vi "sub_updatepos_fgv.vi"(7 "cmd":enum16{"left", "right", "ini", "read", "write"}(ring), 8 "error in":errorcluster, 10 "pos":dbl(slide) scale=-1.0..1.0, 11 "Target":T1={"Position"=0.0, "Invert"=TRUE} {"Position" min=-0.5 max=0.5 step=0.1 format="%.2g"}) -> (0 "error out":errorcluster, 3 "Target_out":T1={"Position"=0.5, "Invert"=FALSE} {"Position" min=-0.5 max=0.5 step=0.1 format="%.2g"})   [LabVIEW 2018]
uses:
  Model/Target.ctl
  Global_val.vi
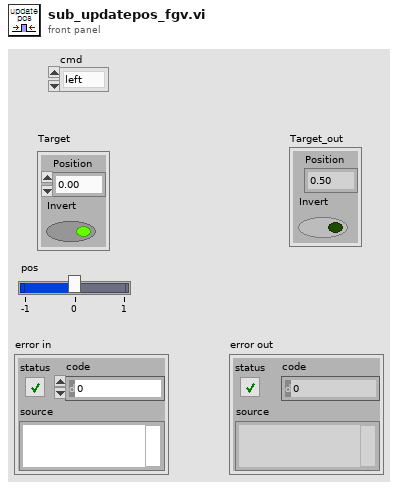
[diagram p1: front panel]
types:
  T1 = typedef "Target.ctl" = cluster{"Position":dbl, "Invert":bool}
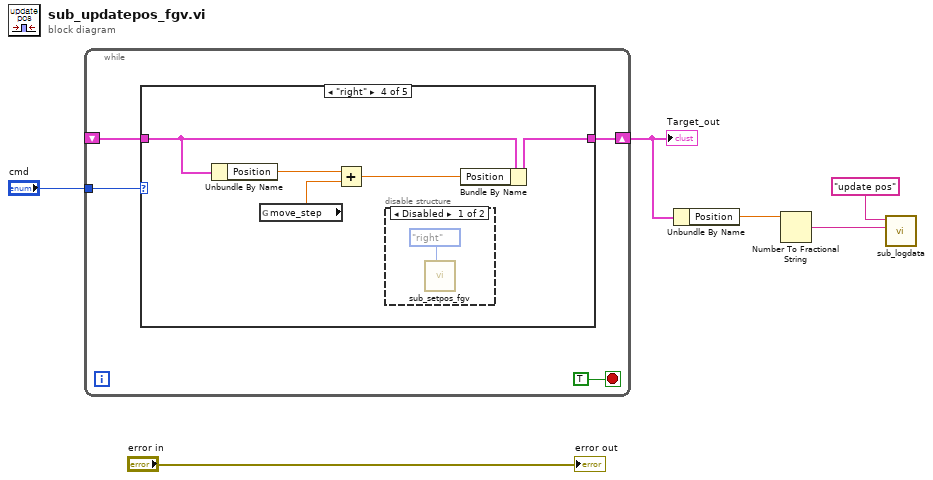
[diagram p0: block diagram]
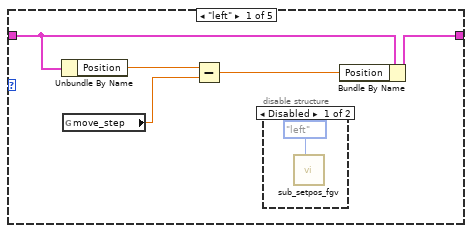
[diagram p2: hidden frame]
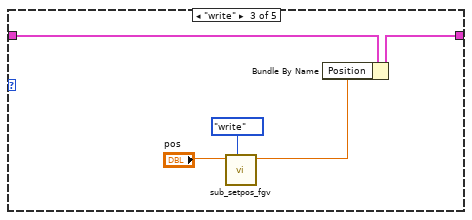
[diagram p5: hidden frame]
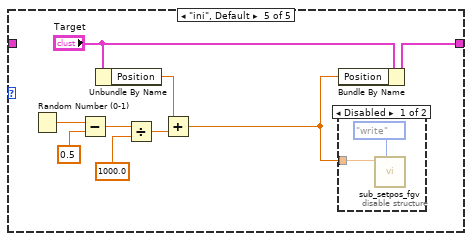
[diagram p7: hidden frame]
diagram:
  n1 = while {
    tunnel: "cmd" -> [w9]
    shift-right: [w8] -> w3
    shift-left: _ -> [w7]
    stop <- TRUE stop-if-true
    n2 = case shown="\"right\"" w9 {
      tunnel: [w15 w17 w20 w27 w33] -> w8
      tunnel: w7 -> [w14 w17 w21 w24 _]
      frame "left" {
        n3 = Unbundle By Name(w14) -> ("Position"=w12:dbl)
        n4 = global read "Global_val.vi" "move_step"() -> (w13:dbl)
        n5 = Subtract(x=w12, y=w13) -> (x-y=w11:dbl)
        n6 = disable-structure shown="Disabled" {
          frame Disabled {
            n7 = call "sub_setpos_fgv.vi"("cmd"=enum16{"read", "init", "left", "write", "right"}."left") -> ()  [unwired: 9 in, 2 out]
          }
          frame Enabled {
          }
        }
        n8 = Bundle By Name(cluster=w14, "Position"=w11) -> (w15:T1)
      }
      frame "read" {
      }
      frame "write" {
        n9 = call "sub_setpos_fgv.vi"("cmd"=enum16{"read", "init", "left", "write", "right"}."write", "Slide"="pos") -> ("set_pos"=w22:dbl)  [unwired: 8 in, 1 out]
        n10 = Bundle By Name(cluster=w21, "Position"=w22) -> (w20:T1)
      }
      frame "right" {
        n11 = Unbundle By Name(w24) -> ("Position"=w25:dbl)
        n12 = global read "Global_val.vi" "move_step"() -> (w26:dbl)
        n13 = Add(x=w25, y=w26) -> (x+y=w23:dbl)
        n14 = disable-structure shown="Disabled" {
          frame Disabled {
            n15 = call "sub_setpos_fgv.vi"("cmd"=enum16{"read", "init", "left", "write", "right"}."right") -> ()  [unwired: 9 in, 2 out]
          }
          frame Enabled {
          }
        }
        n16 = Bundle By Name(cluster=w24, "Position"=w23) -> (w27:T1)
      }
      frame "ini", Default {
        n17 = Random Number (0-1)() -> (number: 0 to 1=w37:dbl)
        n18 = Subtract(x=w37, y=0.5) -> (x-y=w31:dbl)
        n19 = Unbundle By Name("Target") -> ("Position"=w34:dbl)
        n20 = Divide(x=w31, y=1000.0) -> (x/y=w35:dbl)
        n21 = Add(x=w34, y=w35) -> (x+y=w29:dbl)
        n22 = Bundle By Name(cluster="Target", "Position"=w29) -> (w33:T1)
        n23 = disable-structure shown="Disabled" {
          disable-tunnel: w29 -> [w38 _]
          frame Disabled {
            n24 = call "sub_setpos_fgv.vi"("cmd"=enum16{"read", "init", "left", "write", "right"}."write", "Slide"=w38) -> ()  [unwired: 8 in, 2 out]
          }
          frame Enabled {
          }
        }
      }
    }
  }
  "Target_out" <- w3
  n25 = Unbundle By Name(w3) -> ("Position"=w2:dbl)
  n26 = Number To Fractional String(number=w2) -> (F-format string=w1:string)  [unwired: 3 in]
  n27 = call "sub_logdata.vi"("data_str"=w1, "Title"="update pos") -> ()  [unwired: 9 in, 1 out]
  "error out" <- "error in"
